vi "Smista DO.vi"(4 "Forza DO Cdaq":T4, 8 "Forza DO plc 3":T1, 9 "Forza DO plc 2":T2, 10 "Forza DO plc 1":T3, 11 "DO interfaccia in":T5) -> (0 "StatoDO_PLC_3_out":T1, 1 "StatoDO_PLC_2_out":T2, 3 "statoDO Cdaq out":T4)   [LabVIEW 2019]
uses:
  cDAQ_PLC Folder/controls/statoDO_Cdaq.ctl
  TypeDef/DOinterfaccia.ctl
  cDAQ_PLC Folder/ST1200_LIST_IO/StatoDO_PLC_1.ctl
  cDAQ_PLC Folder/ST1200_LIST_IO/StatoDO_PLC_2.ctl
  cDAQ_PLC Folder/ST1200_LIST_IO/StatoDO_PLC_3.ctl
  GlobalForzaUscite.vi
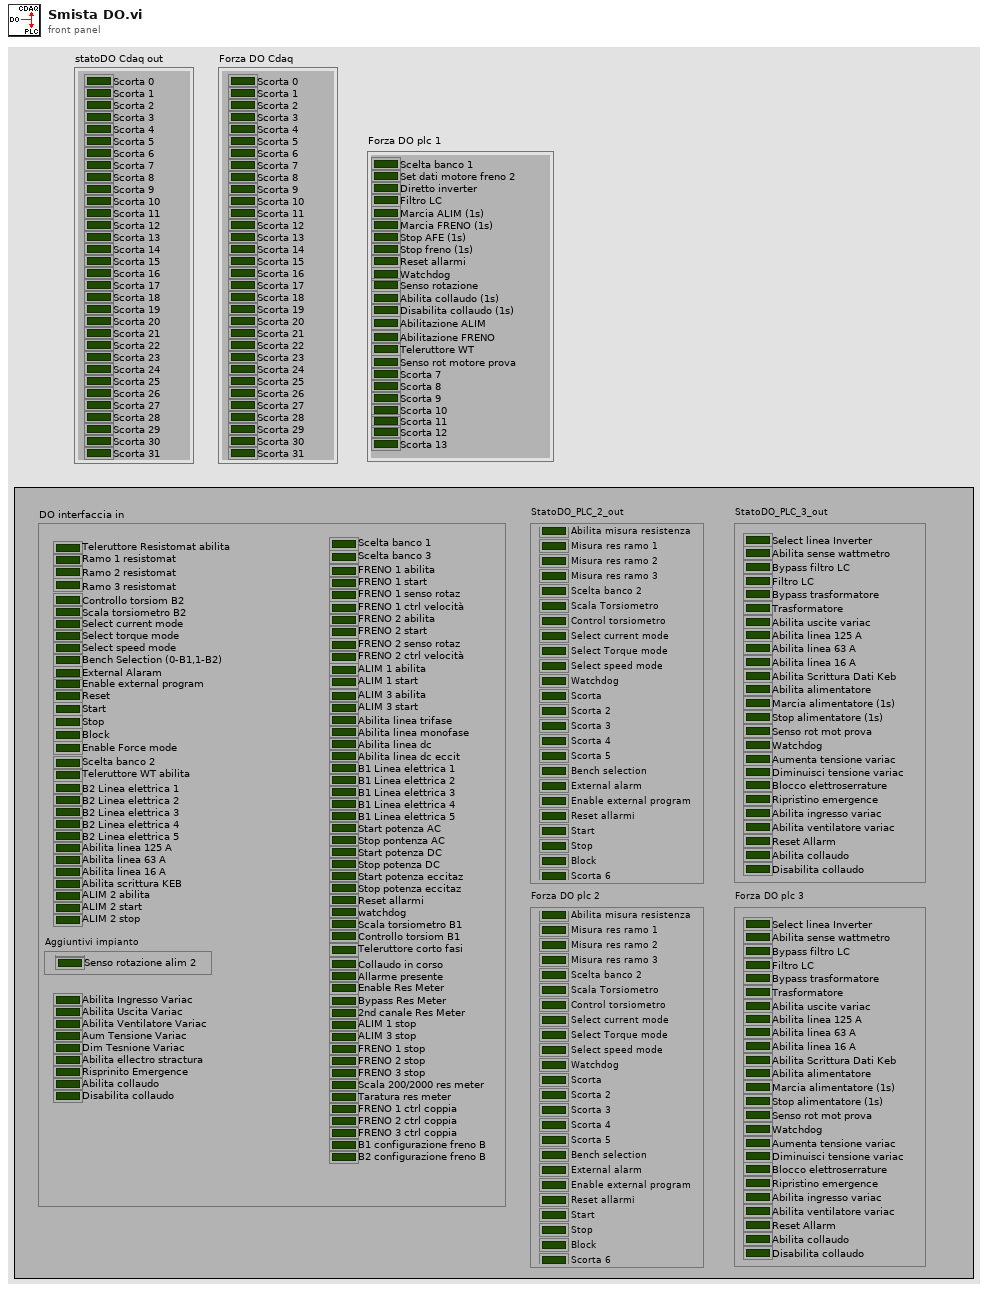
[diagram p1: front panel]
types:
  T1 = typedef "StatoDO_PLC_3.ctl" = cluster{"Select linea Inverter":bool, "Abilita sense wattmetro":bool, "Bypass filtro LC":bool, "Filtro LC":bool, "Bypass trasformatore":bool, "Trasformatore":bool, "Abilita uscite variac":bool, "Abilita linea 125 A":bool, "Abilita linea 63 A":bool, "Abilita linea 16 A":bool, "Abilita Scrittura Dati Keb":bool, "Abilita alimentatore":bool, "Marcia alimentatore (1s)":bool, "Stop alimentatore (1s)":bool, "Senso rot mot prova":bool, "Watchdog":bool, "Aumenta tensione variac":bool, "Diminuisci tensione variac ":bool, "Blocco elettroserrature":bool, "Ripristino emergence":bool, "Abilita ingresso variac":bool, "Abilita ventilatore variac":bool, "Reset Allarm":bool, "Scorta 1":bool, "Scorta 2":bool, "Scorta 3":bool, "Scorta 4":bool, "Scorta 5":bool, "Scorta 6":bool, "Scorta 7":bool, "Scorta 8":bool, "Scorta 9":bool, "Abilita collaudo":bool, "Disabilita collaudo ":bool, "Scorta 10":bool, "Scorta 11":bool, "Scorta 12":bool, "Scorta 13":bool, "Scorta 14":bool, "Scorta 15":bool}
  T2 = typedef "StatoDO_PLC_2.ctl" = cluster{"Relè misura resistomat":bool, "Misura res ramo 1":bool, "Misura res ramo 2":bool, "Misura res ramo 3":bool, "Scelta banco 2":bool, "Scala Torsiometro":bool, "Ctrl torsiometro":bool, "Select current mode":bool, "Select Torque mode":bool, "Select speed mode":bool, "Watchdog":bool, "Scorta":bool, "Scorta 2":bool, "Scorta 3":bool, "Scorta 4":bool, "Scorta 5":bool, "Bench selection":bool, "External alarm":bool, "Enable external program":bool, "Reset allarmi":bool, "Start":bool, "Stop":bool, "Block":bool, "Scorta 6":bool}
  T3 = typedef "StatoDO_PLC_1.ctl" = cluster{"Scelta banco 1":bool, "Set dati motore freno 2":bool, "Diretto inverter":bool, "Filtro LC":bool, "Marcia ALIM (1s)":bool, "Marcia FRENO (1s)":bool, "Stop AFE (1s)":bool, "Stop freno (1s)":bool, "Reset allarmi":bool, "Watchdog":bool, "Senso rotazione":bool, "Abilita collaudo (1s)":bool, "Disabilita collaudo (1s)":bool, "Abilitazione ALIM":bool, "Abilitazione FRENO":bool, "Teleruttore WT":bool, "Senso rot motore prova":bool, "Scorta 7":bool, "Scorta 8":bool, "Scorta 9":bool, "Scorta 10":bool, "Scorta 11":bool, "Scorta 12":bool, "Scorta 13":bool}
  T4 = typedef "statoDO_Cdaq.ctl" = cluster{"Scorta 0":bool, "Scorta 1":bool, "Scorta 2":bool, "Scorta 3":bool, "Scorta 4":bool, "Scorta 5":bool, "Scorta 6":bool, "Scorta 7":bool, "Scorta 8":bool, "Scorta 9":bool, "Scorta 10":bool, "Scorta 11":bool, "Scorta 12":bool, "Scorta 13":bool, "Scorta 14":bool, "Scorta 15":bool, "Scorta 16":bool, "Scorta 17":bool, "Scorta 18":bool, "Scorta 19":bool, "Scorta 20":bool, "Scorta 21":bool, "Scorta 22":bool, "Scorta 23":bool, "Scorta 24":bool, "Scorta 25":bool, "Scorta 26":bool, "Scorta 27":bool, "Scorta 28":bool, "Scorta 29":bool, "Scorta 30":bool, "Scorta 31":bool}
  T5 = typedef "DOinterfaccia.ctl" = cluster{"Scelta banco 1":bool, "Scelta banco 2":bool, "Scelta banco 3":bool, "FRENO 1 abilita":bool, "FRENO 1 start":bool, "FRENO 1 senso rotaz":bool, "FRENO 1 ctrl velocità":bool, "FRENO 2 abilita":bool, "FRENO 2 start":bool, "FRENO 2 senso rotaz":bool, "FRENO 2 ctrl velocità":bool, "ALIM 1 abilita":bool, "ALIM 1 start":bool, "ALIM 2 abilita":bool, "ALIM 2 start":bool, "ALIM 3 abilita":bool, "ALIM 3 start":bool, "Abilita linea trifase":bool, "Abilita linea monofase":bool, "Abilita linea dc":bool, "Abilita linea dc eccit":bool, "B1 Linea elettrica 1":bool, "B1 Linea elettrica 2":bool, "B1 Linea elettrica 3":bool, "B1 Linea elettrica 4":bool, "B1 Linea elettrica 5":bool, "B2 Linea elettrica 1":bool, "B2 Linea elettrica 2":bool, "B2 Linea elettrica 3":bool, "B2 Linea elettrica 4":bool, "B2 Linea elettrica 5":bool, "Start potenza AC":bool, "Stop pontenza AC":bool, "Start potenza DC":bool, "Stop potenza DC":bool, "Start potenza eccitaz":bool, "Stop potenza eccitaz":bool, "Reset allarmi":bool, "watchdog":bool, "Scala torsiometro B1":bool, "Controllo torsiom B1":bool, "Scala torsiometro B2":bool, "Controllo torsiom B2":bool, "Teleruttore WT abilita":bool, "Teleruttore Resistomat abilita":bool, "Teleruttore corto fasi":bool, "Ramo 1 resistomat":bool, "Ramo 2 resistomat":bool, "Ramo 3 resistomat":bool, "Collaudo in corso":bool, "Allarme presente":bool, "Enable Res Meter":bool, "Bypass Res Meter":bool, "2nd canale Res Meter":bool, "Scala 200/2000 res meter":bool, "Taratura res meter":bool, "FRENO 1 ctrl coppia":bool, "FRENO 2 ctrl coppia":bool, "FRENO 3 ctrl coppia":bool, "Aggiuntivi impianto":cluster{"Senso rotazione alim 1":bool, "Senso rotazione alim 2":bool}, "ALIM 1 stop":bool, "ALIM 2 stop":bool, "ALIM 3 stop":bool, "FRENO 1 stop":bool, "FRENO 2 stop":bool, "FRENO 3 stop":bool, "B1 configurazione freno B":bool, "B2 configurazione freno B":bool, "Abilita scrittura KEB":bool, "Bench Selection (0-B1,1-B2)":bool, "Select current mode":bool, "Select torque mode":bool, "Select speed mode":bool, "Start":bool, "Stop":bool, "Block":bool, "Enable Force mode":bool, "Abilita linea 125 A":bool, "Abilita linea 63 A":bool, "Abilita linea 16 A":bool, "Aum Tensione Variac":bool, "Dim Tesnione Variac":bool, "Abilita ellectro stractura":bool, "Risprinito Emergence":bool, "Abilita collaudo":bool, "Disabilita collaudo":bool, "External Alaram":bool, "Enable external program":bool, "Reset":bool, "Abilita Ingresso Variac":bool, "Abilita Ventilatore Variac":bool, "Abilita Uscita Variac ":bool}
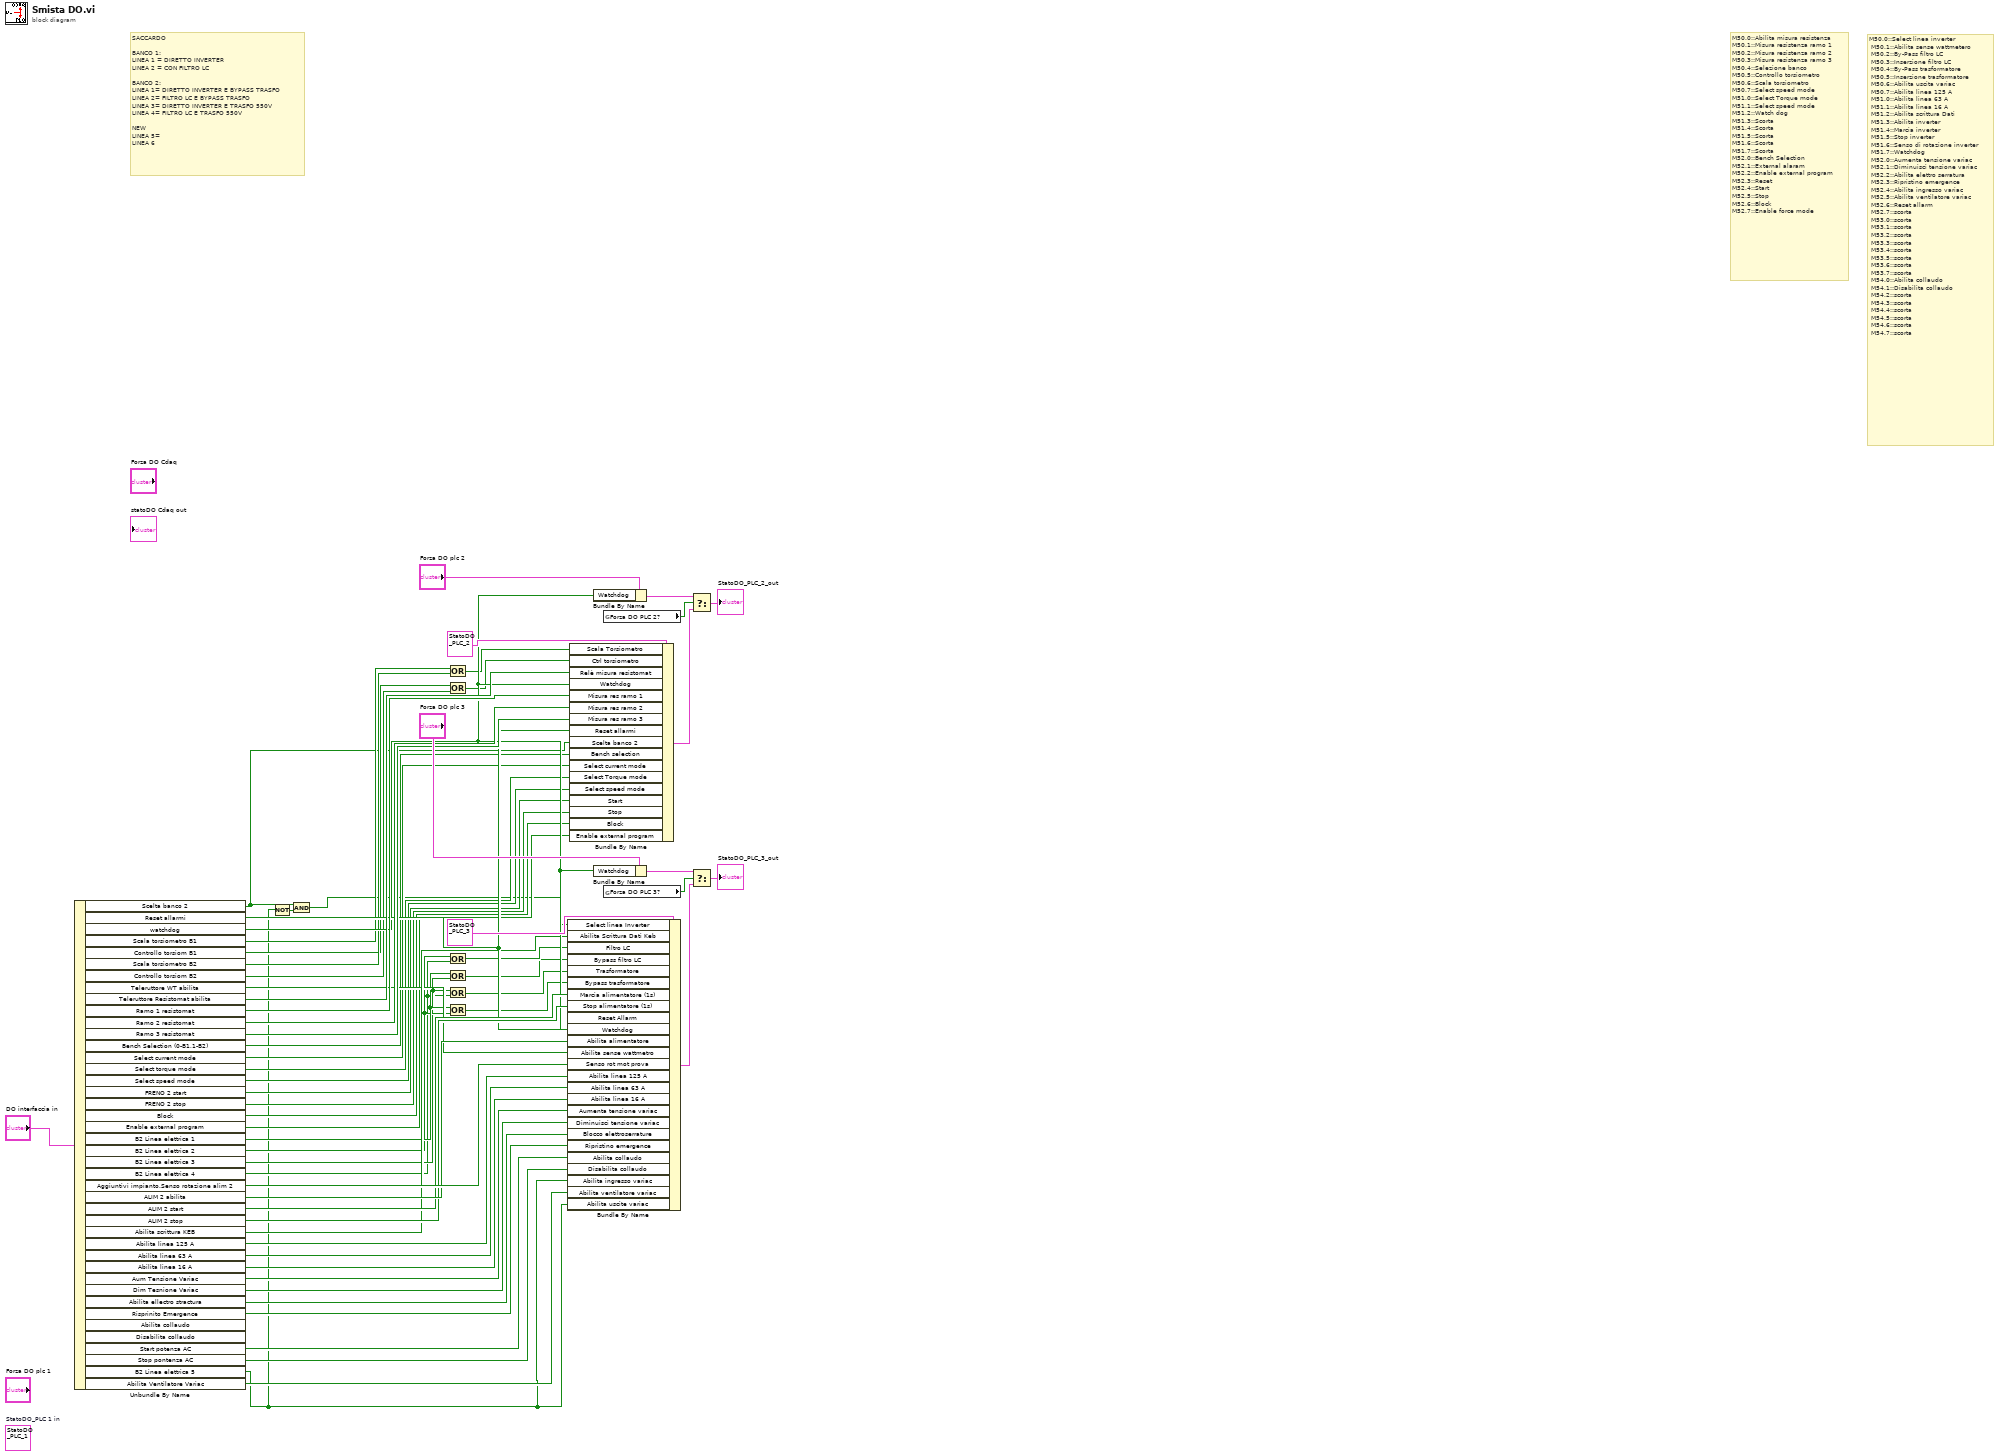
[diagram p0: block diagram]
diagram:
  (unwired) T3 {"Scelta banco 1"=FALSE, "Set dati motore freno 2"=FALSE, "Diretto inverter"=FALSE, "Filtro LC"=FALSE, "Marcia ALIM (1s)"=FALSE, "Marcia FRENO (1s)"=FALSE, "Stop AFE (1s)"=FALSE, "Stop freno (1s)"=FALSE, "Reset allarmi"=FALSE, "Watchdog"=FALSE, "Senso rotazione"=FALSE, "Abilita collaudo (1s)"=FALSE, "Disabilita collaudo (1s)"=FALSE, "Abilitazione ALIM"=FALSE, "Abilitazione FRENO"=FALSE, "Teleruttore WT"=FALSE, "Senso rot motore prova"=FALSE, "Scorta 7"=FALSE, "Scorta 8"=FALSE, "Scorta 9"=FALSE, "Scorta 10"=FALSE, "Scorta 11"=FALSE, "Scorta 12"=FALSE, "Scorta 13"=FALSE}  # StatoDO_PLC 1 in
  # "M50.0::Select linea inverter\n\tM50.1::Abilita sense wattmetero\n\tM50.2::By-Pass filtro LC\n\tM50.3::Inserzione filtro LC\n\tM50.4::By-Pass trasformatore\n\tM50.5::Inserzione trasformatore\n\tM50.6::Abilita uscita variac\n\tM50.7::Abilita linea 125 A\n\tM51.0::Abilita linea 63 A\n\tM51.1::Abilita linea 16 A\n\tM51.2::Abilita scrittura Dati\n\tM51.3::Abilita inverter\n\tM51.4::Marcia inverter\n\tM51.5::Stop inverter\n\tM51.6::Senso di rotazione inverter\n\tM51.7::Watchdog\n\tM52.0::Aumenta tensione variac\n\tM52.1::Diminuisci tensione variac\n\tM52.2::Abilita elettro serratura\n\tM52.3::Ripristino emergence\n\tM52.4::Abilita ingresso variac\n\tM52.5::Abilita ventilatore variac\n\tM52.6::Reset allarm\n\tM52.7::scorta\n\tM53.0::scorta\n\tM53.1::scorta\n\tM53.2::scorta\n\tM53.3::scorta\n\tM53.4::scorta\n\tM53.5::scorta\n\tM53.6::scorta\n\tM53.7::scorta\n\tM54.0::Abilita collaudo\n\tM54.1::Disabilita collaudo\n\tM54.2::scorta\n\tM54.3::scorta\n\tM54.4::scorta\n\tM54.5::scorta\n\tM54.6::scorta\n\tM54.7::scorta"
  # "M50.0::Abilita misura resistenza\nM50.1::Misura resistenza ramo 1\nM50.2::Misura resistenza ramo 2\nM50.3::Misura resistenza ramo 3\nM50.4::Selezione banco\nM50.5::Controllo torsiometro\nM50.6::Scala torsiometro\nM50.7::Select speed mode\nM51.0::Select Torque mode\nM51.1::Select speed mode\nM51.2::Watch dog\nM51.3::Scorta\nM51.4::Scorta\nM51.5::Scorta\nM51.6::Scorta\nM51.7::Scorta\nM52.0::Bench Selection\nM52.1::External alaram\nM52.2::Enable external program\nM52.3::Reset\nM52.4::Start\nM52.5::Stop\nM52.6::Block\nM52.7::Enable force mode"
  # "SACCARDO\n\nBANCO 1:\nLINEA 1 = DIRETTO INVERTER\nLINEA 2 = CON FILTRO LC\n\nBANCO 2:\nLINEA 1= DIRETTO INVERTER E BYPASS TRASFO\nLINEA 2= FILTRO LC E BYPASS TRASFO\nLINEA 3= DIRETTO INVERTER E TRASFO 550V\nLINEA 4= FILTRO LC E TRASFO 550V\n\nNEW\nLINEA 5=\nLINEA 6"
  n1 = Unbundle By Name("DO interfaccia in") -> ("Scelta banco 2"=w2:bool, "Reset allarmi"=w40:bool, "watchdog"=w39:bool, "Scala torsiometro B1"=w32:bool, "Controllo torsiom B1"=w30:bool, "Scala torsiometro B2"=w33:bool, "Controllo torsiom B2"=w29:bool, "Teleruttore WT abilita"=w27:bool, "Teleruttore Resistomat abilita"=w49:bool, "Ramo 1 resistomat"=w48:bool, "Ramo 2 resistomat"=w47:bool, "Ramo 3 resistomat"=w46:bool, "Bench Selection (0-B1,1-B2)"=w26:bool, "Select current mode"=w18:bool, "Select torque mode"=w17:bool, "Select speed mode"=w16:bool, "FRENO 2 start"=w15:bool, "FRENO 2 stop"=w14:bool, "Block"=w13:bool, "Enable external program"=w12:bool, "B2 Linea elettrica 1"=w11:bool, "B2 Linea elettrica 2"=w10:bool, "B2 Linea elettrica 3"=w9:bool, "B2 Linea elettrica 4"=w8:bool, "Aggiuntivi impianto.Senso rotazione alim 2"=w44:bool, "ALIM 2 abilita"=w43:bool, "ALIM 2 start"=w42:bool, "ALIM 2 stop"=w41:bool, "Abilita scrittura KEB"=w34:bool, "Abilita linea 125 A"=w25:bool, "Abilita linea 63 A"=w24:bool, "Abilita linea 16 A"=w23:bool, "Aum Tensione Variac"=w22:bool, "Dim Tesnione Variac"=w21:bool, "Abilita ellectro stractura"=w20:bool, "Risprinito Emergence"=w19:bool, "Start potenza AC"=w7:bool, "Stop pontenza AC"=w6:bool, "B2 Linea elettrica 5"=w1:bool, "Abilita Ventilatore Variac"=w5:bool)  [unwired: 2 out]
  n2 = Not(x=w1) -> (.not. x?=w4:bool)
  n3 = And(x=w2, y=w4) -> (x .and. y?=w3:bool)
  n4 = Or(x=w32, y=w33) -> (x .or. y?=w31:bool)
  n5 = Or(x=w30, y=w29) -> (x .or. y?=w28:bool)
  n6 = Or(x=w10, y=w8) -> (x .or. y?=w37:bool)
  n7 = Or(x=w11, y=w9) -> (x .or. y?=w35:bool)
  n8 = Or(x=w9, y=w8) -> (x .or. y?=w36:bool)
  n9 = Or(x=w11, y=w10) -> (x .or. y?=w38:bool)
  n10 = Bundle By Name(cluster=T1 {"Select linea Inverter"=FALSE, "Abilita sense wattmetro"=FALSE, "Bypass filtro LC"=FALSE, "Filtro LC"=FALSE, "Bypass trasformatore"=FALSE, "Trasformatore"=FALSE, "Abilita uscite variac"=FALSE, "Abilita linea 125 A"=FALSE, "Abilita linea 63 A"=FALSE, "Abilita linea 16 A"=FALSE, "Abilita Scrittura Dati Keb"=FALSE, "Abilita alimentatore"=FALSE, "Marcia alimentatore (1s)"=FALSE, "Stop alimentatore (1s)"=FALSE, "Senso rot mot prova"=FALSE, "Watchdog"=FALSE, "Aumenta tensione variac"=FALSE, "Diminuisci tensione variac "=FALSE, "Blocco elettroserrature"=FALSE, "Ripristino emergence"=FALSE, "Abilita ingresso variac"=FALSE, "Abilita ventilatore variac"=FALSE, "Reset Allarm"=FALSE, "Scorta 1"=FALSE, "Scorta 2"=FALSE, "Scorta 3"=FALSE, "Scorta 4"=FALSE, "Scorta 5"=FALSE, "Scorta 6"=FALSE, "Scorta 7"=FALSE, "Scorta 8"=FALSE, "Scorta 9"=FALSE, "Abilita collaudo"=FALSE, "Disabilita collaudo "=FALSE, "Scorta 10"=FALSE, "Scorta 11"=FALSE, "Scorta 12"=FALSE, "Scorta 13"=FALSE, "Scorta 14"=FALSE, "Scorta 15"=FALSE} ("StatoDO_PLC_3_out"), "Select linea Inverter"=w3, "Abilita Scrittura Dati Keb"=w34, "Filtro LC"=w37, "Bypass filtro LC"=w35, "Trasformatore"=w36, "Bypass trasformatore"=w38, "Marcia alimentatore (1s)"=w42, "Stop alimentatore (1s)"=w41, "Reset Allarm"=w40, "Watchdog"=w39, "Abilita alimentatore"=w43, "Abilita sense wattmetro"=w27, "Senso rot mot prova"=w44, "Abilita linea 125 A"=w25, "Abilita linea 63 A"=w24, "Abilita linea 16 A"=w23, "Aumenta tensione variac"=w22, "Diminuisci tensione variac"=w21, "Blocco elettroserrature"=w20, "Ripristino emergence"=w19, "Abilita collaudo"=w7, "Disabilita collaudo"=w6, "Abilita ingresso variac"=w1, "Abilita ventilatore variac"=w5, "Abilita uscite variac"=w1) -> (w55:T1)
  n11 = Bundle By Name(cluster=T2 {"Relè misura resistomat"=FALSE, "Misura res ramo 1"=FALSE, "Misura res ramo 2"=FALSE, "Misura res ramo 3"=FALSE, "Scelta banco 2"=FALSE, "Scala Torsiometro"=FALSE, "Ctrl torsiometro"=FALSE, "Select current mode"=FALSE, "Select Torque mode"=FALSE, "Select speed mode"=FALSE, "Watchdog"=FALSE, "Scorta"=FALSE, "Scorta 2"=FALSE, "Scorta 3"=FALSE, "Scorta 4"=FALSE, "Scorta 5"=FALSE, "Bench selection"=FALSE, "External alarm"=FALSE, "Enable external program"=FALSE, "Reset allarmi"=FALSE, "Start"=FALSE, "Stop"=FALSE, "Block"=FALSE, "Scorta 6"=FALSE} ("StatoDO_PLC_2_out"), "Scala Torsiometro"=w31, "Ctrl torsiometro"=w28, "Relè misura resistomat"=w49, "Watchdog"=w39, "Misura res ramo 1"=w48, "Misura res ramo 2"=w47, "Misura res ramo 3"=w46, "Reset allarmi"=w40, "Scelta banco 2"=w2, "Bench selection"=w26, "Select current mode"=w18, "Select Torque mode"=w17, "Select speed mode"=w16, "Start"=w15, "Stop"=w14, "Block"=w13, "Enable external program"=w12) -> (w56:T2)
  n12 = Bundle By Name(cluster="Forza DO plc 2", "Watchdog"=w39) -> (w53:T2)
  n13 = Bundle By Name(cluster="Forza DO plc 3", "Watchdog"=w39) -> (w51:T1)
  n14 = global read "GlobalForzaUscite.vi" "Forza DO PLC 2?"() -> (w60:bool)
  n15 = global read "GlobalForzaUscite.vi" "Forza DO PLC 3?"() -> (w58:bool)
  n16 = Select(t=w53, s=w60, f=w56) -> (s? t:f=→"StatoDO_PLC_2_out":T2)
  n17 = Select(t=w51, s=w58, f=w55) -> (s? t:f=→"StatoDO_PLC_3_out":T1)
